vi "PM100D_Meas_NPLC.vi"(9 "Command":string, 10 "NCPL":i32=1, 11 "VISA Refnum in":refnum<visa-resource-name>) -> (2 "Array":dbl[](array[numeric]), 3 "Error":bool, 4 "Value":string, 5 "INF":u32)   [LabVIEW 2011]
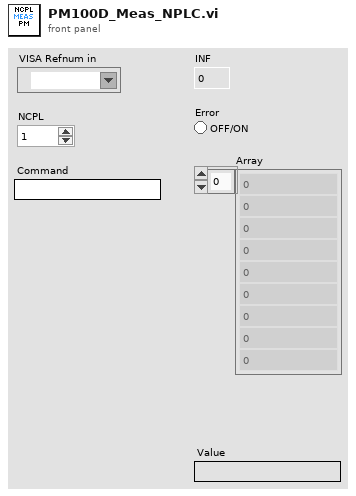
[diagram p1: front panel]
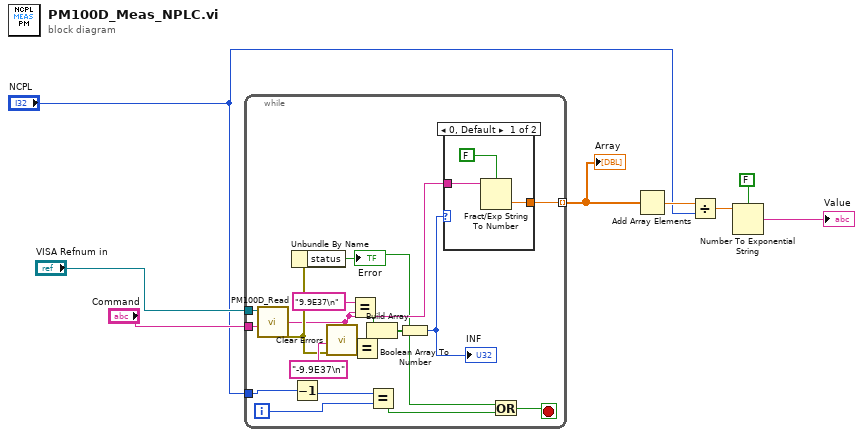
[diagram p0: block diagram]
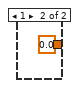
[diagram p2: hidden frame]
diagram:
  n1 = while {
    tunnel: "VISA Refnum in" -> [w25]
    tunnel: "Command" -> [w24]
    tunnel: [w15] -> w4 mode=indexing
    tunnel: "NCPL" -> [w10]
    i -> [w11]
    stop <- w14 stop-if-true
    n2 = call "PM100D_Read.vi"("Command"=w24, "VISA in"=w25) -> ("error out"=w18:errorcluster, "ReadValue"=w17:string)  [unwired: 2 in, 1 out]
    n3 = Unbundle By Name(w18) -> ("status"=w12:bool)
    "Error" <- w12
    n4 = Decrement(x=w10) -> (x-1=w9:i32)
    n5 = call <vilib>:"Clear Errors.vi"("error in (no error)"=w18) -> ()  [unwired: 6 in, 1 out]
    n6 = Equal?(x="9.9E37\n", y=w17) -> (x = y?=w20:bool)
    n7 = Equal?(x="-9.9E37\n", y=w17) -> (x = y?=w21:bool)
    n8 = Build Array(w20, w21) -> (w19:bool[])
    n9 = Equal?(x=w9, y=w11) -> (x = y?=w13:bool)
    n10 = Boolean Array To Number(Boolean array=w19) -> (number=w16:u32)
    "INF" <- w16
    n11 = case shown="0, Default" w16 {
      tunnel: w17 -> [w27 _]
      tunnel: [w26 0.0] -> w15
      frame 0, Default {
        n12 = Fract/Exp String To Number(use system decimal point (T)=FALSE, string=w27) -> (number=w26:dbl)  [unwired: 2 in, 1 out]
      }
      frame 1 {
      }
    }
    n13 = Or(x=w12, y=w13) -> (x .or. y?=w14:bool)
  }
  "Array" <- w4
  n14 = Add Array Elements(numeric array=w4) -> (sum=w5:dbl)
  n15 = Divide(x=w5, y="NCPL") -> (x/y=w6:dbl)
  n16 = Number To Exponential String(number=w6, 1:FALSE ("use system decimal point (T)")) -> (E-format string=→"Value":string)  [unwired: 2 in]
